vi "Transliterate String.vi"(0 "text in":string, 1 "map":u8[](array[numeric])) -> (2 "text out":string)   [LabVIEW 2015, in "Car Wash.lvlib" / "Tools_String.lvlib"]
doc: "Maps characters in \"text in\" according to \"map\".\n\nIf \"map\" is an array of 256 elements, then\n\n text_out[i] = map[ text_in[i] ]\n\notherwise\n\n text_out[i] = text_i [i]"
uses:
  Tools_String.lvlib
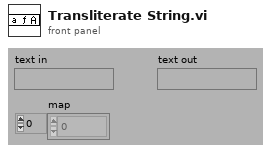
[diagram p1: front panel]
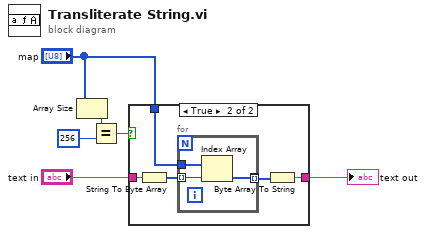
[diagram p0: block diagram]
diagram:
  n1 = Array Size(array="map") -> (size(s)=w4:i32)
  n2 = Equal?(x=w4, y=256) -> (x = y?=w1:bool)
  n3 = case shown="True" w1 {
    tunnel: [w7 w12] -> w5
    tunnel: "text in" -> [w7 w10]
    tunnel: "map" -> [_ w9]
    frame False {
    }
    frame True {
      n4 = String To Byte Array(string=w10) -> (unsigned byte array=w11:u8[])
      n5 = for {
        tunnel: w11 -> [w15] mode=indexing
        tunnel: [w14] -> _ mode=indexing
        tunnel: w9 -> [w13]
        tunnel: [w14] -> w8 mode=indexing
        n6 = Index Array(array=w13, index=w15) -> (element=w14:u8)
      }
      n7 = Byte Array To String(unsigned byte array=w8) -> (string=w12:string)
    }
  }
  "text out" <- w5
